vi "aoc-2025-d02-2.vi"() -> ()   [LabVIEW 2020]
panel:
  out "numbers with patterns":u64[](array[numeric])
  out "sum":u64
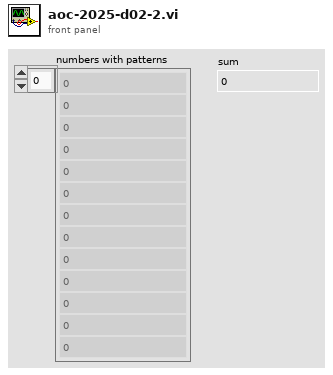
[diagram p1: front panel]
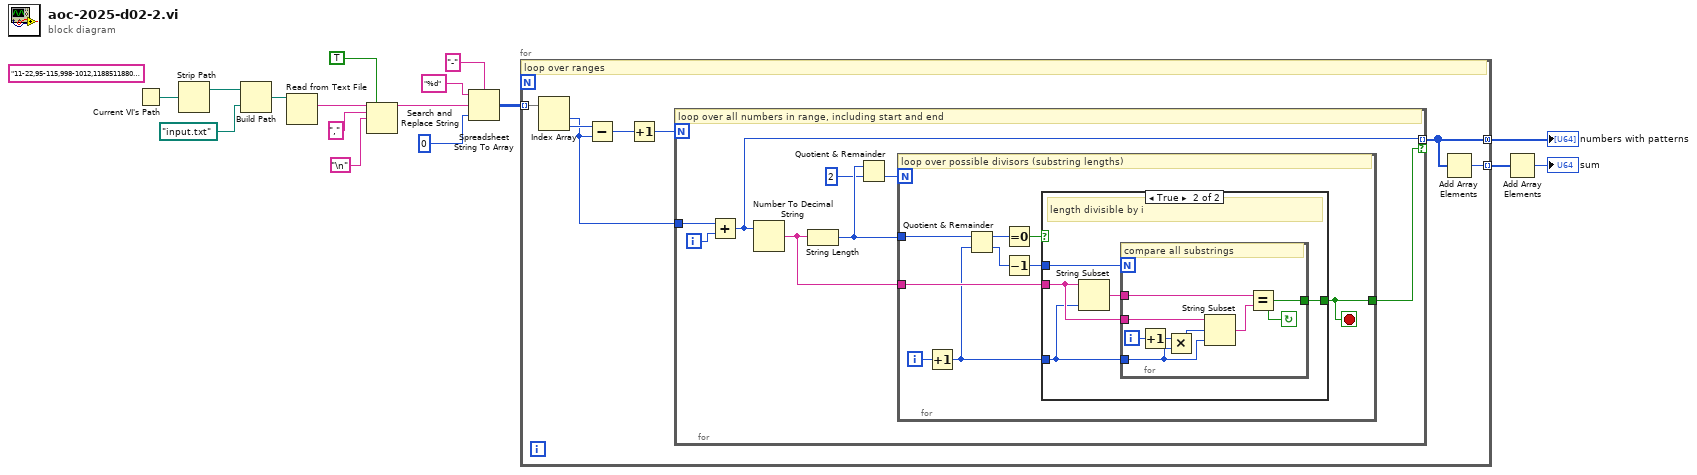
[diagram p0: block diagram]
diagram:
  (unwired) "11-22,95-115,998-1012,1188511880-1188511890,222220-222224,1698522-1698528,446443-446449,38593856-38593862,565653-565659,824824821-824824827,2121212118-2121212124" ("input string")
  n1 = Current VI's Path() -> (path=w6:path)
  n2 = Strip Path(path=w6) -> (stripped path=w5:path)  [unwired: 1 out]
  n3 = Build Path(base path=w5, name or relative path=path "input.txt") -> (appended path=w3:path)
  n4 = Read from Text File(file (use dialog)=w3) -> (text=w1:string)  [unwired: 3 in, 3 out]
  n5 = Search and Replace String(replace all?=TRUE ("replace all? (F)"), input string=w1, search string=",", replace string="\n") -> (result string=w10:string)  [unwired: 4 in, 3 out]
  n6 = Spreadsheet String To Array(delimiter (Tab)="-", format string="%d", spreadsheet string=w10, array type (2D Dbl)=u64 0) -> (array=w9:u64[][])
  n7 = for {
    tunnel: w9 -> [w23] mode=indexing
    tunnel: [w18] -> w8 mode=indexing
    tunnel: [w17] -> w2 mode=concatenating
    # "loop over ranges"
    n8 = Index Array(array=w23) -> (element #1=w20:u64, element #2=w22:u64)  [unwired: 2 in]
    n9 = Subtract(x=w22, y=w20) -> (x-y=w21:u64)
    n10 = Increment(x=w21) -> (x+1=w19:u64)
    n11 = for {
      N: w19 -> [_]
      tunnel: w20 -> [w31]
      tunnel: [w28] -> w17 mode=indexing if=w27
      i -> [w30]
      # "loop over all numbers in range, including start and end"
      n12 = Add(x=w31, y=w30) -> (x+y=w28:u64)
      n13 = Number To Decimal String(number=w28) -> (decimal integer string=w29:string)  [unwired: 1 in]
      n14 = String Length(string=w29) -> (length=w26:i32)
      n15 = Quotient & Remainder(x=w26, y=2) -> (floor(x/y)=w25:i32)  [unwired: 1 out]
      n16 = for {
        N: w25 -> [_]
        tunnel: w29 -> [w38]
        tunnel: [w32] -> w27
        tunnel: w26 -> [w37]
        i -> [w36]
        stop <- w32 stop-if-true
        # "loop over possible divisors (substring lengths)"
        n17 = Increment(x=w36) -> (x+1=w34:i32)
        n18 = Quotient & Remainder(x=w37, y=w34) -> (x-y*floor(x/y)=w40:i32, floor(x/y)=w35:i32)
        n19 = Equal To 0?(x=w40) -> (x = 0?=w39:bool)
        n20 = Decrement(x=w35) -> (x-1=w33:i32)
        n21 = case shown="True" w39 {
          tunnel: w38 -> [_ w45]
          tunnel: w34 -> [_ w44]
          tunnel: [_ w42] -> w32
          tunnel: w33 -> [_ w41]
          frame False {
          }
          frame True {
            # "length divisible by i"
            n22 = String Subset(string=w45, length (rest)=w44) -> (substring=w43:string)  [unwired: 1 in]
            n23 = for {
              N: w41 -> [_]
              tunnel: w45 -> [w53]
              tunnel: w44 -> [w50]
              tunnel: w43 -> [w48]
              tunnel: [w47] -> w42
              i -> [w52]
              stop <- w47 continue-if-true
              # "compare all substrings"
              n24 = Increment(x=w52) -> (x+1=w46:i32)
              n25 = Multiply(x=w46, y=w50) -> (x*y=w51:i32)
              n26 = String Subset(string=w53, offset (0)=w51, length (rest)=w50) -> (substring=w49:string)
              n27 = Equal?(x=w48, y=w49) -> (x = y?=w47:bool)
            }
          }
        }
      }
    }
    n28 = Add Array Elements(numeric array=w17) -> (sum=w18:u64)
  }
  "numbers with patterns" <- w2
  n29 = Add Array Elements(numeric array=w8) -> (sum=→"sum":u64)
